vi "placementHandler.vi"(4 "NewVal":bool, 5 "Enum":enum16{"Player 1 Turn", "Player 2 Turn"}(ring), 6 "AllObjs[]":refnum<vi>[](array[refnum]), 7 "Array":T2(array[cluster]), 9 "Array 3":cluster{u32, u32}[](array[cluster]), 10 "Array 2":T1(array[cluster]), 11 "Boolean in":refnum<vi>) -> (0 "error out":errorcluster, 1 "numTrue":i32, 3 "x":enum16{"Player 1 Turn", "Player 2 Turn"}(ring))   [LabVIEW 2014]
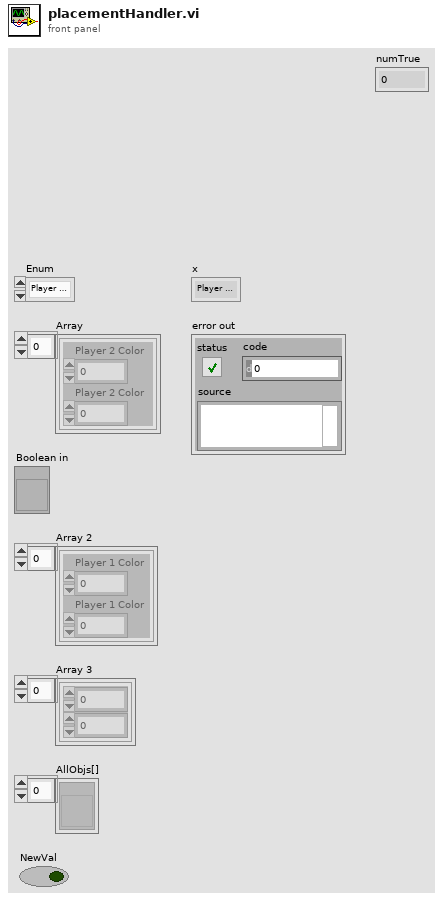
[diagram p1: front panel]
types:
  T1 = cluster{"Player 1 Color":u32, "Player 1 Color":u32}[]
  T2 = cluster{"Player 2 Color ":u32, "Player 2 Color ":u32}[]
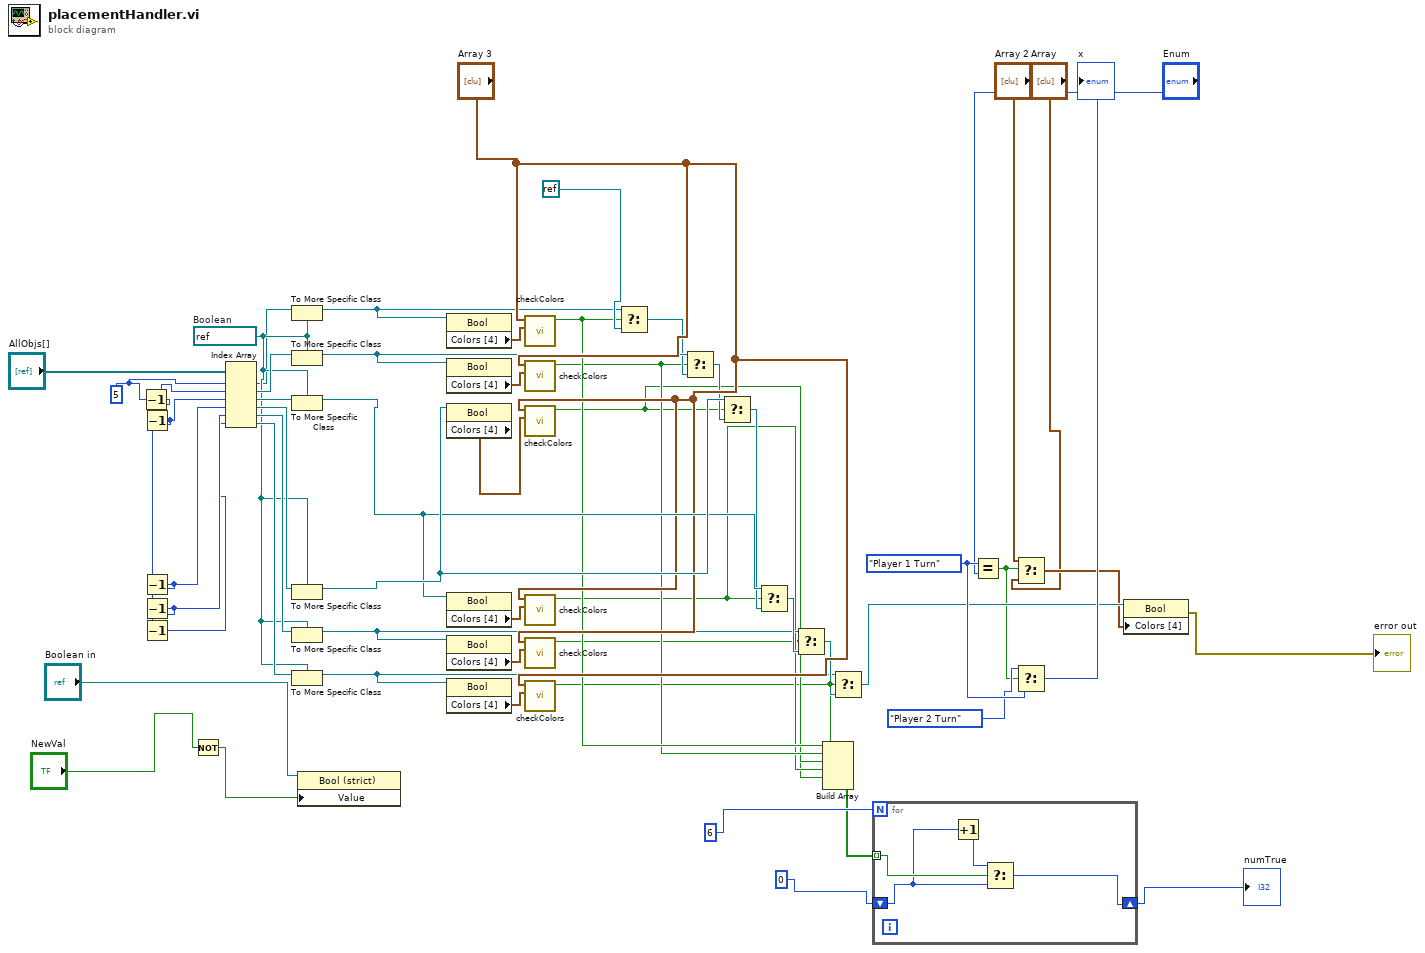
[diagram p0: block diagram]
diagram:
  w56 = enum16{"Player 1 Turn", "Player 2 Turn"}."Player 1 Turn" ("x")
  w18 = refnum<vi> refnum  # Boolean
  w12 = 5
  n1 = Decrement(x=w12) -> (x-1=w14:i32)
  n2 = Decrement(x=w14) -> (x-1=w15:i32)
  n3 = Decrement(x=w15) -> (x-1=w16:i32)
  n4 = Decrement(x=w16) -> (x-1=w17:i32)
  n5 = Decrement(x=w17) -> (x-1=w13:i32)
  n6 = Not(x="NewVal") -> (.not. x?=w46:bool)
  n7 = Index Array(array="AllObjs[]", index #1=w12, index #2=w14, index #3=w15, index #4=w16, index #5=w17, index #6=w13) -> (element #1=w11:refnum<vi>, element #2=w19:refnum<vi>, element #3=w20:refnum<vi>, element #4=w21:refnum<vi>, element #5=w22:refnum<vi>, element #6=w23:refnum<vi>)
  n8 = To More Specific Class(target class=w18, reference=w11) -> (specific class reference=w37:refnum<vi>)  [unwired: 1 in, 1 out]
  n9 = To More Specific Class(target class=w18, reference=w19) -> (specific class reference=w38:refnum<vi>)  [unwired: 1 in, 1 out]
  n10 = To More Specific Class(target class=w18, reference=w20) -> (specific class reference=w42:refnum<vi>)  [unwired: 1 in, 1 out]
  n11 = To More Specific Class(target class=w18, reference=w21) -> (specific class reference=w43:refnum<vi>)  [unwired: 1 in, 1 out]
  n12 = To More Specific Class(target class=w18, reference=w22) -> (specific class reference=w31:refnum<vi>)  [unwired: 1 in, 1 out]
  n13 = To More Specific Class(target class=w18, reference=w23) -> (specific class reference=w30:refnum<vi>)  [unwired: 1 in, 1 out]
  n14 = property class="Bool (strict)"(reference="Boolean in", "Value"=w46) -> ()  [unwired: 1 in, 2 out]
  n15 = property class="Bool"(reference=w37) -> ("Colors [4]"=w24:cluster{u32, u32}[])  [unwired: 1 in, 2 out]
  n16 = property class="Bool"(reference=w38) -> ("Colors [4]"=w25:cluster{u32, u32}[])  [unwired: 1 in, 2 out]
  n17 = property class="Bool"(reference=w43) -> ("Colors [4]"=w26:cluster{u32, u32}[])  [unwired: 1 in, 2 out]
  n18 = property class="Bool"(reference=w42) -> ("Colors [4]"=w27:cluster{u32, u32}[])  [unwired: 1 in, 2 out]
  n19 = property class="Bool"(reference=w31) -> ("Colors [4]"=w28:cluster{u32, u32}[])  [unwired: 1 in, 2 out]
  n20 = property class="Bool"(reference=w30) -> ("Colors [4]"=w29:cluster{u32, u32}[])  [unwired: 1 in, 2 out]
  n21 = call "checkColors.vi"("Colors [4]"=w24, "Array"="Array 3") -> ("Boolean"=w9:bool)  [unwired: 9 in]
  n22 = call "checkColors.vi"("Colors [4]"=w25, "Array"="Array 3") -> ("Boolean"=w8:bool)  [unwired: 9 in]
  n23 = call "checkColors.vi"("Colors [4]"=w26, "Array"="Array 3") -> ("Boolean"=w7:bool)  [unwired: 9 in]
  n24 = call "checkColors.vi"("Colors [4]"=w27, "Array"="Array 3") -> ("Boolean"=w6:bool)  [unwired: 9 in]
  n25 = call "checkColors.vi"("Colors [4]"=w28, "Array"="Array 3") -> ("Boolean"=w5:bool)  [unwired: 9 in]
  n26 = call "checkColors.vi"("Colors [4]"=w29, "Array"="Array 3") -> ("Boolean"=w4:bool)  [unwired: 9 in]
  n27 = Select(t=w37, s=w9, f=refnum<k0> refnum) -> (s? t:f=w36:refnum<vi>)
  n28 = Select(t=w38, s=w8, f=w36) -> (s? t:f=w35:refnum<vi>)
  n29 = Select(t=w43, s=w7, f=w35) -> (s? t:f=w34:refnum<vi>)
  n30 = Select(t=w42, s=w6, f=w34) -> (s? t:f=w33:refnum<vi>)
  n31 = Select(t=w31, s=w5, f=w33) -> (s? t:f=w32:refnum<vi>)
  n32 = Build Array(w9, w8, w7, w6, w5, w4) -> (w3:bool[])
  n33 = Select(t=w30, s=w4, f=w32) -> (s? t:f=w52:refnum<vi>)
  n34 = for {
    N: 6 -> [_]
    tunnel: w3 -> [w59] mode=indexing
    shift-right: [w57] -> w1
    shift-left: 0 -> [w58]
    n35 = Increment(x=w58) -> (x+1=w60:i32)
    n36 = Select(t=w60, s=w59, f=w58) -> (s? t:f=w57:i32)
  }
  "numTrue" <- w1
  n37 = Equal?(x=w56, y="Enum") -> (x = y?=w51:bool)
  n38 = Select(t="Array 2", s=w51, f="Array") -> (s? t:f=w50:T2)
  n39 = Select(t=enum16{"Player 1 Turn", "Player 2 Turn"}."Player 2 Turn" ("x"), s=w51, f=w56) -> (s? t:f=→"x":enum16{"Player 1 Turn", "Player 2 Turn"})
  n40 = property class="Bool"(reference=w52, "Colors [4]"=w50) -> (error out=→"error out":errorcluster)  [unwired: 1 in, 1 out]
